vi "Configure Reference Levels [WM].vi"(0 "CS++Scope":refnum<class "CS++Scope.lvclass">, 5 "low reference (10.0%)":dbl=10.0 format="%.3f", 7 "mid reference (50.0%)":dbl=50.0 format="%.3f", 9 "high reference (90.0%)":dbl=90.0 format="%.3f", 11 "error in (no error)":errorcluster) -> (4 "CS++Scope out":refnum<class "CS++Scope.lvclass">, 15 "error out":errorcluster)   [LabVIEW 2016, in "CS++Scope.lvlib" / "CS++Scope.lvclass"]
doc: "This VI configures the reference levels for waveform measurements. \n\nYou must call this VI before you call the IviScope Read Waveform Measurement [WM] or IviScope Fetch Waveform Measurement [WM] to take a rise time, fall time, width negative, width positive, duty cycle negative, duty cycle positive, preshoot, or overshoot measurement.\n\nNotes:\n\n(1) This VI is part of the IviScopeWaveformMeasurement [WM] extension group."
uses:
  CS++Scope.lvclass
  CSPP_Core/Classes/CS++ProcessVariables/ProcessVariable/PV.lvclass
  PV-Enum.ctl
  CS++Scope.lvclass/CS++Scope.ctl
  CSPP_Core/Classes/CS++ProcessVariables/ProcessVariable/PV.lvclass/PV.ctl
  CSPP_Core/Classes/CS++ProcessVariables/ProcessVariable/Write Data.vi
  CSPP_Core/Classes/CS++ProcessVariables/ProcessVariable/Write Timestamp.vi
  CSPP_Core/Classes/CS++ProcessVariables/ProcessVariable/Write Quality.vi
  CSPP_Core/Classes/CS++ProcessVariables/ProcessVariable/Write status.vi
  CSPP_Core/Classes/CS++ProcessVariables/PVConnection/PVConnection.lvclass
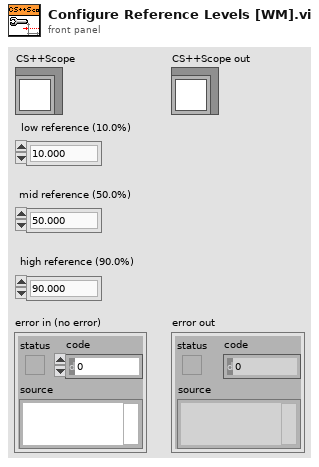
[diagram p1: front panel]
types:
  T1 = typedef "CS++Scope.lvlib/CS++Scope.lvclass/PV-Enum.ctl" = enum16{"ActualSampleRate", "TimePerRecord", "AcquisitionStartTime", "TriggerLevel", "GlitchWidth", "LowReference", "MidReference", "HighReference", "RuntLowThreshold", "RuntHighThreshold", "TriggerHoldoff", "WidthLowThreshold", "WidthHighThreshold", "AcquisitionStatus", "ActualRecordLength", "ActualSampleMode", "ACLineTriggerSlope", "MinRecordLength", "AcquisitionType", "TriggerSlope", "GlitchCondition", "GlitchPolarity", "InterpolationMethod", "NumberOfAverages", "NumberOfEnvelopes", "TriggerType", "TriggerCoupling", "TriggerModifier", "TVLineNumber", "TVEvent", "TVTriggerPolarity", "TVSignalFormat", "WidthCondition", "WidthPolarity", "MeasurementDone", "ContinousAcquisition", "TriggerSource", "Waveform", "ActualTimeIncrement"}
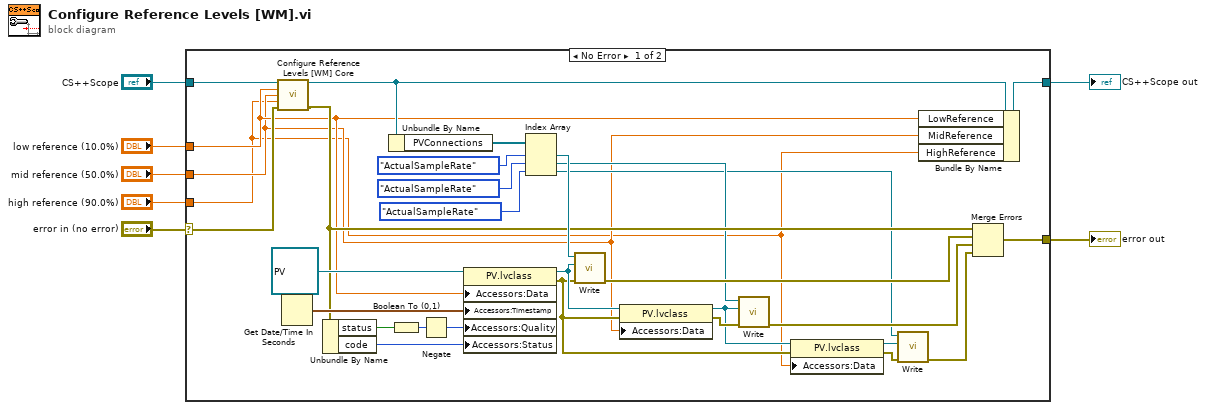
[diagram p0: block diagram]
diagram:
  n1 = case shown="No Error" "error in (no error)" {
    selector: "error in (no error)" -> [w12 w40]
    tunnel: [w11 w40] -> w6
    tunnel: [w13 w39] -> w2
    tunnel: "CS++Scope" -> [w14 w39]
    tunnel: "low reference (10.0%)" -> [w10 _]
    tunnel: "mid reference (50.0%)" -> [w9 _]
    tunnel: "high reference (90.0%)" -> [w8 _]
    frame No Error {
      n2 = call-dynamic "Configure Reference Levels [WM] Core.vi"("CS++Scope"=w14, "low reference (10.0%)"=w10, "mid reference (50.0%)"=w9, "high reference (90.0%)"=w8, "error in (no error)"=w12) -> ("CS++Scope out"=w28:refnum<class "CS++Scope.lvclass">, "error out"=w27:errorcluster)  [unwired: 9 in]
      n3 = Get Date/Time In Seconds() -> (seconds since 1Jan1904=w33:timestamp)
      n4 = Unbundle By Name(w27) -> ("status"=w36:bool, "code"=w37:i32)
      n5 = Unbundle By Name(w28) -> ("PVConnections"=w32:refnum<class "PVConnection.lvclass">[])
      n6 = Boolean To (0,1)(Boolean=w36) -> (0, 1=w35:i16)
      n7 = Negate(x=w35) -> (-x=w34:i16)
      n8 = property class="PV.lvclass"(reference=refnum<class "PV.lvclass"> refnum ("CS++ProcessVariables.lvlib:PV.lvclass"), "Accessors:Data"=w10, "Accessors:Timestamp"=w33, "Accessors:Quality"=w34, "Accessors:Status"=w37) -> (reference out=w22:refnum<class "PV.lvclass">, error out=w18:errorcluster)  [unwired: 1 in]
      n9 = Index Array(array=w32, index #1=PV-Enum."ActualSampleRate" ("PV-Enum"), index #2=PV-Enum."ActualSampleRate" ("PV-Enum"), index #3=PV-Enum."ActualSampleRate" ("PV-Enum")) -> (element #1=w30:refnum<class "PVConnection.lvclass">, element #2=w20:refnum<class "PVConnection.lvclass">, element #3=w16:refnum<class "PVConnection.lvclass">)
      n10 = call "Write.vi"("error in (no error)"=w18, "PV"=w22, "PVConnection in"=w30) -> ("error out"=w29:errorcluster)  [unwired: 7 in, 1 out]
      n11 = property class="PV.lvclass"(reference=w22, error in=w18, "Accessors:Data"=w9) -> (reference out=w19:refnum<class "PV.lvclass">, error out=w21:errorcluster)
      n12 = call "Write.vi"("error in (no error)"=w21, "PV"=w19, "PVConnection in"=w20) -> ("error out"=w24:errorcluster)  [unwired: 7 in, 1 out]
      n13 = property class="PV.lvclass"(reference=w19, error in=w18, "Accessors:Data"=w8) -> (reference out=w17:refnum<class "PV.lvclass">, error out=w15:errorcluster)
      n14 = call "Write.vi"("error in (no error)"=w15, "PV"=w17, "PVConnection in"=w16) -> ("error out"=w23:errorcluster)  [unwired: 7 in, 1 out]
      n15 = Bundle By Name(cluster=w28, "LowReference"=w10, "MidReference"=w9, "HighReference"=w8) -> (w13:refnum<class "CS++Scope.lvclass">)
      n16 = Merge Errors(w27, w29, w24, w23) -> (w11:errorcluster)
    }
    frame Error {
    }
  }
  "error out" <- w6
  "CS++Scope out" <- w2
